vi "Toggle3.vi"(1 "In":bool) -> (0 "Out":bool)   [LabVIEW 2011]
panel:
  in  "Start Toggling":bool
  in  "InternalValue":bool
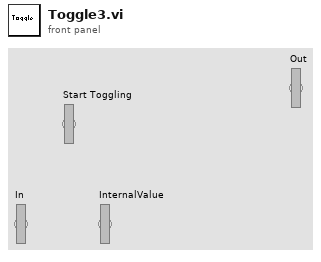
[diagram p1: front panel]
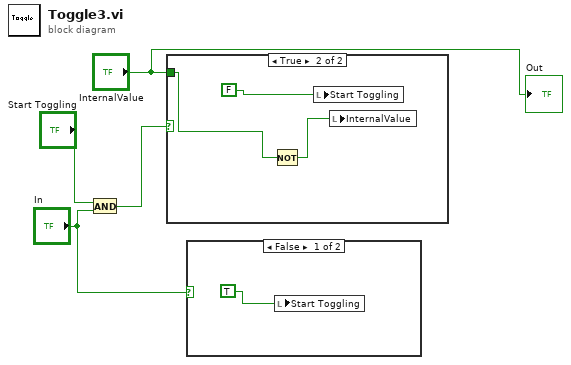
[diagram p0: block diagram]
diagram:
  n1 = And(x="Start Toggling", y="In") -> (x .and. y?=w4:bool)
  n2 = case shown="True" w4 {
    tunnel: "InternalValue" -> [_ w5]
    frame False {
    }
    frame True {
      n3 = Not(x=w5) -> (.not. x?=w6:bool)
      n4 = local write "Start Toggling"(FALSE) -> ()
      n5 = local write "InternalValue"(w6) -> ()
    }
  }
  n6 = case shown="False" "In" {
    frame False {
      n7 = local write "Start Toggling"(TRUE) -> ()
    }
    frame True {
    }
  }
  "Out" <- "InternalValue"
